vi "proj1.vi"() -> ()   [LabVIEW 2023]
panel:
  in  "stop":bool
  in  "Amplituda":dbl
  out "Waveform Chart":dynamicdata(graph)
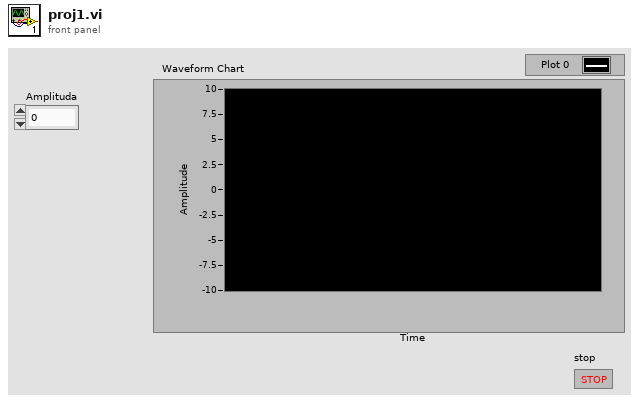
[diagram p1: front panel]
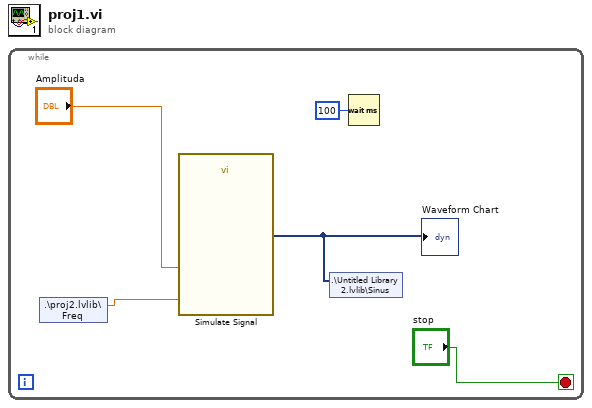
[diagram p0: block diagram]
diagram:
  n1 = while {
    stop <- "stop" stop-if-true
    n2 = shared-variable ".\\proj2.lvlib\\Freq"() -> (w3:dbl)  [unwired: 1 in, 1 out]
    n3 = call "Simulate Signal"("Frequency"=w3, "Amplitude"="Amplituda") -> ("Sine"=w2:dynamicdata)  [unwired: 12 in, 1 out]
    "Waveform Chart" <- w2
    n4 = shared-variable ".\\Untitled Library 2.lvlib\\Sinus"(w2) -> ()  [unwired: 1 in, 1 out]
    n5 = Wait (ms)(milliseconds to wait=u32 100) -> ()  [unwired: 1 out]
  }
